vi "TSCAN_LoadCANDBC.vi"(8 "error in (no error)":errorcluster, 9 "ABindChannels":i32[](array[ring])=[0] items=["CHN1", "CHN2", "CHN3", "CHN4", "CHN5", "CHN6", "CHN7", "CHN8", "CHN9", "CHN10", "CHN11", "CHN12", "CHN13", "CHN14", "CHN15", "CHN16", "CHN17", "CHN18", "CHN19", "CHN20", "CHN21", "CHN22", "CHN23", "CHN24", "CHN25", "CHN26", "CHN27", "CHN28", "CHN29", "CHN30", "CHN31", "CHN32"], 10 "ADBCAbsolutePath":path=path "C:/Users/DYR/Desktop/M110.dbc", 11 "Path":path) -> (0 "error out":errorcluster, 1 "AIdOut":u32, 2 "return":i32, 3 "Path output":path)   [LabVIEW 2014]
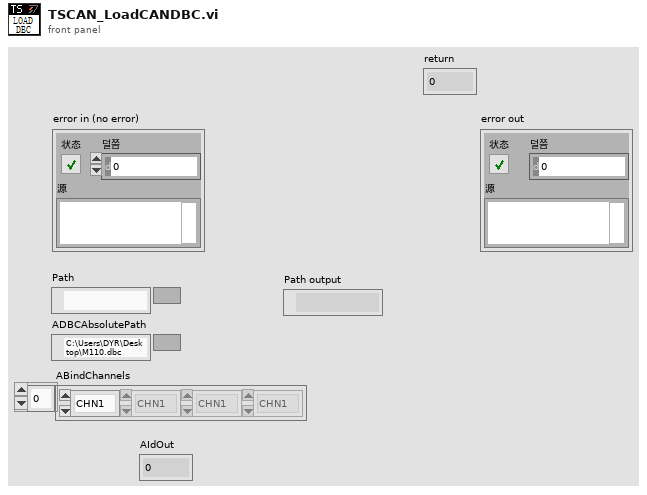
[diagram p1: front panel]
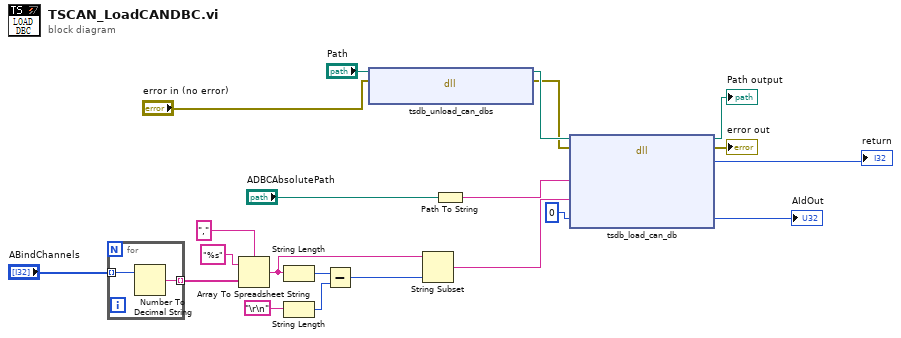
[diagram p0: block diagram]
diagram:
  n1 = for {
    tunnel: "ABindChannels" -> [w23] mode=indexing
    tunnel: [w22] -> w6 mode=indexing
    n2 = Number To Decimal String(number=w23) -> (decimal integer string=w22:string)  [unwired: 1 in]
  }
  n3 = Array To Spreadsheet String(delimiter (Tab)="," ("delimiter"), array=w6, 3:"%s" ("format string")) -> (spreadsheet string=w8:string)
  n4 = String Length(string=w8) -> (length=w10:i32)
  n5 = String Length(string="\r\n") -> (length=w9:i32)
  n6 = Subtract(x=w10, y=w9) -> (x-y=w7:i32)
  n7 = dll-call lib="PTH27abs EDemo同星\nTSCAN_V1.0ConfigTSMaster.dll" fn="tsdb_unload_can_dbs"(path in="Path", error in="error in (no error)") -> (path out=w13:path, error out=w1:errorcluster)  [unwired: 2 in]
  n8 = String Subset(string=w8, length (rest)=w7) -> (substring=w4:string)  [unwired: 1 in]
  n9 = Path To String(path="ADBCAbsolutePath") -> (string=w19:string)
  n10 = dll-call lib="PTH27abs EDemo同星\nTSCAN_V1.0ConfigTSMaster.dll" fn="tsdb_load_can_db"(path in=w13, error in=w1, "ADBCAbsolutePath"=w19, "ABindChannels"=w4, "AId"=u32 0 ("AIdIn")) -> (path out=→"Path output":path, error out=→"error out":errorcluster, "tsdb_load_can_db"=→"return":i32, "AId"=→"AIdOut":i32)  [unwired: 3 in]
